vi "To Pythonic - String.vi"(4 "String":string) -> (1 "Pythonic Value":string)   [LabVIEW 2012, in "OPI.lvclass"]
doc: "Convert LabVIEW data into valid pythonic representation."
uses:
  OPI.lvclass
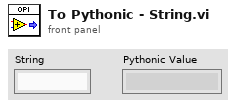
[diagram p1: front panel]
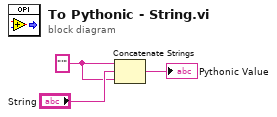
[diagram p0: block diagram]
diagram:
  w1 = "'" ("string")
  n1 = Concatenate Strings(w1, "String", w1) -> (→"Pythonic Value":string)
